vi "OmegaKernel.vi"(11 "Ch Description":T1 {"Duty" format="%016b"; "D" format="%#_5g"; "C" format="%#_5g"; "B" format="%#_5g"; "A" format="%#_5g"}) -> (3 "Reading":dbl)   [LabVIEW 2017]
uses:
  ADAM Client/Sub VIs/ADAM Controls/Ch_description_ADAM.ctl
  ADAM Client/Sub VIs/ADAM Controls/Module_type_ADAM.ctl
  ADAM Client/Sub VIs/ADAM Controls/Function_ADAM.ctl
  ADAM Client/Sub VIs/ADAM Controls/Channel_State.ctl
  ADAM Client/Sub VIs/ADAM Controls/Calib_type_ADAM.ctl
  ADAM Client/Sub VIs/ADAM Controls/Address.ctl
  ADAM Client/Sub VIs/ADAM Controls/Remember_value_mode.ctl
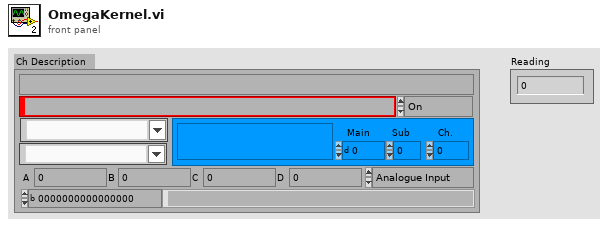
[diagram p1: front panel]
types:
  T1 = typedef "Ch_description_ADAM.ctl" = cluster{"Ch Name":string, "Type":T2, "Function":T3, "Ch State":T4, "Calibration type":T5, "A":dbl, "B":dbl, "C":dbl, "D":dbl, "Comments":string, "Address":T6, "String":string, "Duty":u16}
  T2 = typedef "Module_type_ADAM.ctl" = string
  T3 = typedef "Function_ADAM.ctl" = enum16{"Analogue Input", "Digital Input", "Event counter", "Event rate", "Analogue Output", "Digital Output", "Relay Output"}
  T4 = typedef "Channel_State.ctl" = enum16{"On", "Off", "Always On", "Always Off"}
  T5 = typedef "Calib_type_ADAM.ctl" = string
  T6 = typedef "Address.ctl" = cluster{"Main":i32, "Ch.":i32, "Sub":i32, "Port Name":string}
  T7 = typedef "Remember_value_mode.ctl" = enum16{"Read only", "Read and Write"}
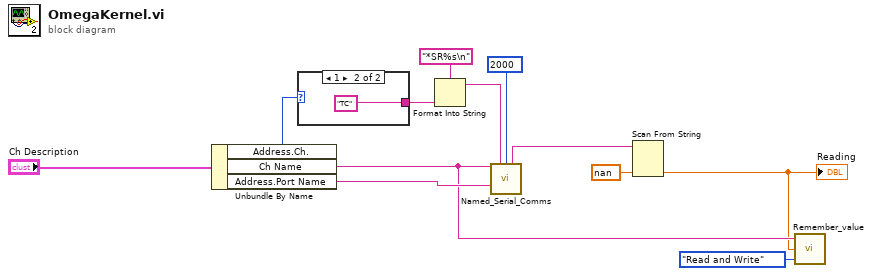
[diagram p0: block diagram]
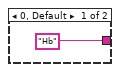
[diagram p2: hidden frame]
diagram:
  n1 = Unbundle By Name("Ch Description") -> ("Address.Ch."=w9:i32, "Ch Name"=w3:string, "Address.Port Name"=w5:string)
  n2 = case shown="1" w9 {
    tunnel: ["Hb" "TC"] -> w11
    frame 0, Default {
    }
    frame 1 {
    }
  }
  n3 = Format Into String(format string="*SR%s\n", w11) -> (resulting string=w10:string)  [unwired: 2 in, 1 out]
  n4 = call "Named_Serial_Comms.vi"("Channel Name"=w3, "Write"=w10, "Timeout/ms"=u32 2000, "Port Name"=w5) -> ("Read"=w8:string)  [unwired: 8 in, 3 out]
  n5 = Scan From String(input string=w8, default 1=nan ("default value 1")) -> (output 1=w2:dbl)  [unwired: 3 in, 3 out]
  "Reading" <- w2
  n6 = call "Remember_value.vi"("Mode"=Remember_value_mode."Read and Write", "Input Value"=w2, "Ch name"=w3) -> ()  [unwired: 1 out]
